vi "add_pose_stamped.vi"(3 "frame_id":string, 4 "Pose":T1, 5 "msg in":string) -> (2 "msg out":string)   [LabVIEW 2015]
doc: "Flattens a stamped pose into a string"
panel:
  in  "reset seq?":bool
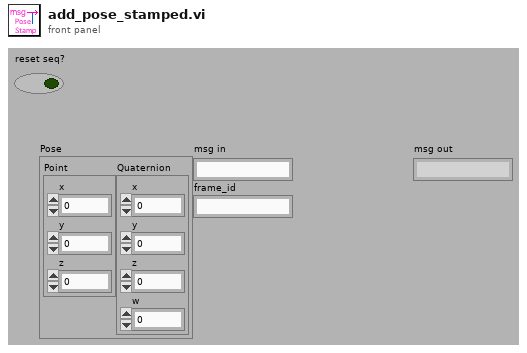
[diagram p1: front panel]
types:
  T1 = cluster{"Point":cluster{"x":dbl, "y":dbl, "z":dbl}, "Quaternion":cluster{"x":dbl, "y":dbl, "z":dbl, "w":dbl}}
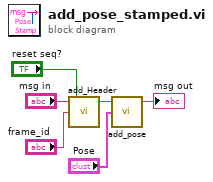
[diagram p0: block diagram]
diagram:
  n1 = call "add_Header.vi"("reset seq?"="reset seq?", "frame_id"="frame_id", "msg in"="msg in") -> ("msg out"=w6:string)  [unwired: 2 in]
  n2 = call "add_pose.vi"("Pose"="Pose", "msg in"=w6) -> ("msg out"=→"msg out":string)  [unwired: 3 in]
